vi "ConvertBytesToBase64.vi"(11 "U8 array":u8[](array[numeric])) -> (3 "base64 encoded":string)   [LabVIEW 2017]
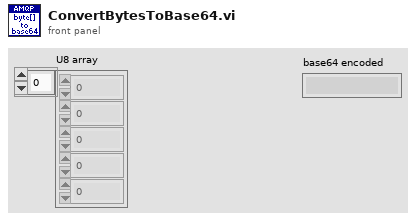
[diagram p1: front panel]
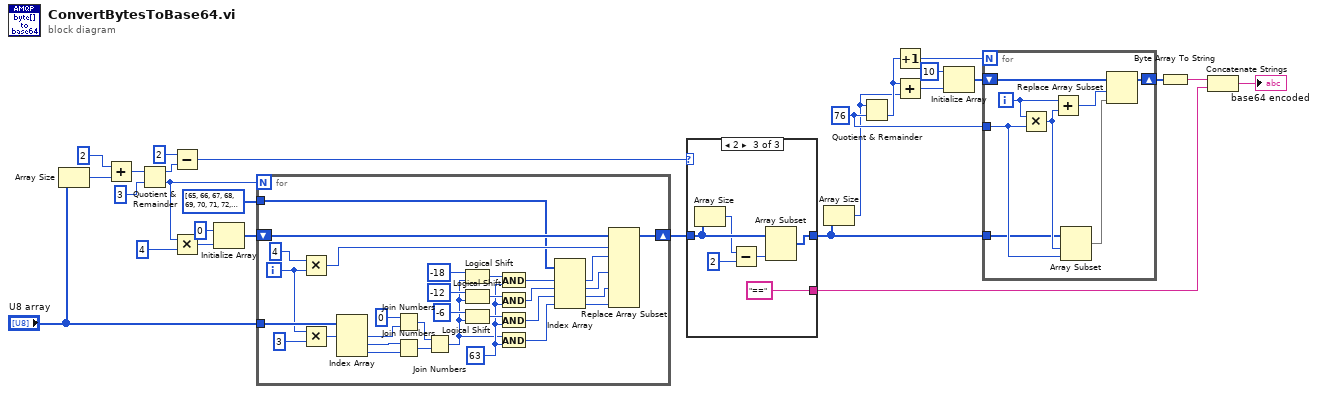
[diagram p0: block diagram]
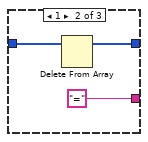
[diagram p3: hidden frame]
diagram:
  w4 = 76 ("y")
  n1 = Array Size(array="U8 array") -> (size(s)=w20:i32)
  n2 = Add(x=2 ("y"), y=w20) -> (x+y=w26:i32)
  n3 = Quotient & Remainder(x=w26, y=3) -> (x-y*floor(x/y)=w24:i32, floor(x/y)=w13:i32)
  n4 = Subtract(x=2, y=w24) -> (x-y=w22:i32)
  n5 = Multiply(x=w13, y=4) -> (x*y=w2:i32)
  n6 = Initialize Array(u8 0 ("Numeric"), w2) -> (w14:u8[])
  n7 = for {
    N: w13 -> [_]
    shift-right: [w36] -> w16
    shift-left: w14 -> [w37]
    tunnel: "U8 array" -> [w58]
    tunnel: u8[] [65, 66, 67, 68, 69, 70, 71, 72, 73, 74, 75, 76, 77, 78, 79, 80, 81, 82, 83, 84, 85, 86, 87, 88, 89, 90, 97, 98, 99, 100, 101, 102, 103, 104, 105, 106, 107, 108, 109, 110, 111, 112, 113, 114, 115, 116, 117, 118, 119, 120, 121, 122, 48, 49, 50, 51, 52, 53, 54, 55, 56, 57, 43, 47] ("unsigned byte array") -> [w28]
    i -> [w35]
    w43 = u32 63
    n8 = Multiply(x=4, y=w35) -> (x*y=w33:i32)
    n9 = Multiply(x=w35, y=3 ("x")) -> (x*y=w50:i32)
    n10 = Index Array(array=w58, index #1=w50) -> (element #1=w41:u8, element #2=w40:u8, element #3=w39:u8)  [unwired: 2 in]
    n11 = Join Numbers(hi=u8 0 ("lo"), lo=w41) -> ((hi.lo)=w49:u16)
    n12 = Join Numbers(hi=w40, lo=w39) -> ((hi.lo)=w48:u16)
    n13 = Join Numbers(hi=w49, lo=w48) -> ((hi.lo)=w38:u32)
    n14 = Logical Shift(y=i8 -18, x=w38) -> (x << y=w56:u32)
    n15 = Logical Shift(y=i8 -12, x=w38) -> (x << y=w55:u32)
    n16 = Logical Shift(y=i8 -6, x=w38) -> (x << y=w46:u32)
    n17 = And(x=w56, y=w43) -> (x .and. y?=w52:u32)
    n18 = And(x=w55, y=w43) -> (x .and. y?=w45:u32)
    n19 = And(x=w46, y=w43) -> (x .and. y?=w44:u32)
    n20 = And(x=w38, y=w43) -> (x .and. y?=w51:u32)
    n21 = Index Array(array=w28, index #1=w52, index #2=w45, index #3=w44, index #4=w51) -> (element #1=w32:u8, element #2=w31:u8, element #3=w30:u8, element #4=w29:u8)
    n22 = Replace Array Subset(array=w37, new element #1=w32, index #1=w33, new element #2=w31, new element #3=w30, new element #4=w29) -> (w36:u8[])  [unwired: 3 in]
  }
  n23 = case shown="2" w22 {
    tunnel: [_ "=" "=="] -> w18
    tunnel: [w59 w60 w67] -> w3
    tunnel: w16 -> [w59 w61 w66]
    frame 0, Default {
    }
    frame 1 {
      n24 = Delete From Array(array=w61) -> (array with subset deleted=w60:u8[])  [unwired: 2 in, 1 out]
    }
    frame 2 {
      n25 = Array Size(array=w66) -> (size(s)=w65:i32)
      n26 = Subtract(x=w65, y=2) -> (x-y=w63:i32)
      n27 = Array Subset(array=w66, length=w63) -> (w67:u8[])  [unwired: 1 in]
    }
  }
  n28 = Array Size(array=w3) -> (size(s)=w1:i32)
  n29 = Quotient & Remainder(x=w1, y=w4) -> (floor(x/y)=w6:i32)  [unwired: 1 out]
  n30 = Increment(x=w6) -> (x+1=w7:i32)
  n31 = Add(x=w6, y=w1) -> (x+y=w10:i32)
  n32 = Initialize Array(u8 10 ("Numeric"), w10) -> (w9:u8[])
  n33 = for {
    N: w7 -> [_]
    shift-right: [w76] -> w5
    shift-left: w9 -> [w70]
    tunnel: w4 -> [w71]
    tunnel: w3 -> [w69]
    i -> [w73]
    n34 = Multiply(x=w73, y=w71) -> (x*y=w74:i32)
    n35 = Add(x=w73, y=w74) -> (x+y=w72:i32)
    n36 = Array Subset(array=w69, index=w74, length=w71) -> (w75:u8[])
    n37 = Replace Array Subset(array=w70, new element=w75, index=w72) -> (w76:u8[])
  }
  n38 = Byte Array To String(unsigned byte array=w5) -> (string=w19:string)
  n39 = Concatenate Strings(w19, w18) -> (→"base64 encoded":string)
